vi "N6700_Initialize.vi"(0 "Instrument Info":T1, 1 "User Reference":i32, 5 "error in (no error)":errorcluster) -> (19 "error out":errorcluster)   [LabVIEW 2018, in "N6700.lvclass"]
uses:
  N6700.lvclass
  Station/Station Support/Controls/Instrument Info.ctl
  C:/Users/John Gmitter/OneDrive - National Instruments/Git Repo/Harris-FL/Reference Management Server/Instrument Drivers/Power_Supply/Power_Supply Virtual/Power_Supply Virtual.lvclass
  N6700.lvclass/N6700.ctl
  Power_Supply Virtual/Power_Supply Virtual.lvclass
  <instrlib>/Agilent N6700 Series/Agilent N6700 Series.lvlib
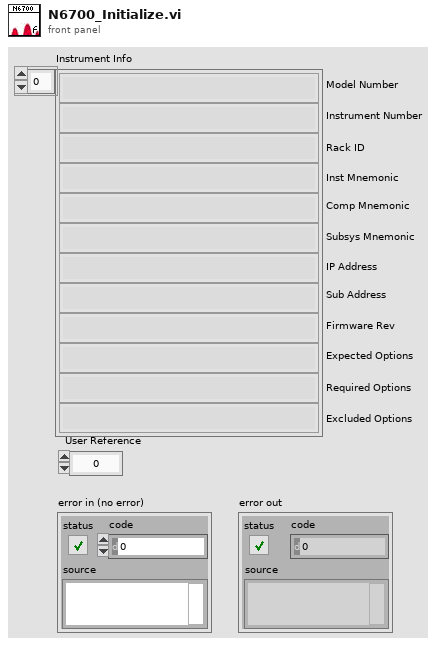
[diagram p1: front panel]
types:
  T1 = typedef "Instrument Info.ctl" = string[]
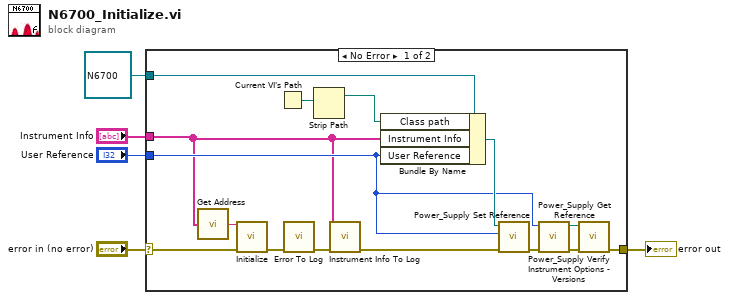
[diagram p0: block diagram]
diagram:
  n1 = case shown="No Error" "error in (no error)" {
    selector: "error in (no error)" -> [w11 w21]
    tunnel: [w16 w21] -> w4
    tunnel: "Instrument Info" -> [w8 _]
    tunnel: "User Reference" -> [w18 _]
    tunnel: refnum<class "N6700.lvclass"> refnum ("N6702A.lvclass") -> [w12 _]
    frame No Error {
      n2 = call "Get Address.vi"("Instrument Info"=w8) -> ("Address"=w9:string)  [unwired: 4 in]
      n3 = call <instrlib>:"Initialize.vi"("VISA resource name"=w9, "error in (no error)"=w11) -> ("error out"=w10:errorcluster)  [unwired: 12 in, 1 out]
      n4 = Current VI's Path() -> (path=w7:path)
      n5 = call "Error To Log.vi"("error in (no error)"=w10) -> ("error out"=w13:errorcluster)  [unwired: 14 in]
      n6 = Strip Path(path=w7) -> (stripped path=w6:path)  [unwired: 1 out]
      n7 = call "Instrument Info To Log.vi"("Instrument Info"=w8, "error in (no error)"=w13) -> ("error out"=w14:errorcluster)  [unwired: 13 in]
      n8 = Bundle By Name(cluster=w12, "Class path"=w6, "Instrument Info"=w8, "User Reference"=w18) -> (w20:refnum<class "N6700.lvclass">)
      n9 = call "Power_Supply Set Reference.vi"("error in (no error)"=w14, "User Reference"=w18, "Power_Supply Virtual.lvclass"=w20) -> ("error out"=w19:errorcluster)  [unwired: 8 in]
      n10 = call "Power_Supply Get Reference.vi"("error in (no error)"=w19, "Instrument Reference"=w18) -> ("error out"=w17:errorcluster, "Power_Supply Virtual.lvclass"=w15:refnum<class "Power_Supply Virtual.lvclass">)  [unwired: 7 in, 1 out]
      n11 = call-dynamic "Power_Supply Verify Instrument Options - Versions.vi"("error in (no error)"=w17, "Power_Supply Virtual in"=w15) -> ("error out"=w16:errorcluster)  [unwired: 8 in, 1 out]
    }
    frame Error {
    }
  }
  "error out" <- w4
